vi "LDVLinearStage.vi"() -> ()   [LabVIEW 2016]
uses:
  <vilib>/Instr/_visa.llb/VISA Configure Serial Port (Instr).vi
panel:
  out "Response":string
  in  "Stop":bool
  in  "Starting Distance (mm)":dbl
  in  "Total Distance (mm)":dbl
  in  "Change in Distance (mm)":dbl
  in  "Wait Time (s)":u32
  in  "Send Commands":bool
  in  "Extra Commands":string
  # "Relevant SCL Commands\n\nAC - Acceleration\nFL - Feed to Length\nFP - Feed to Position\nID - Immediate Distance\nIP - Immediate Position\nJS - Jog Speed\nSJ - Stop Jogging\nSK - Stop and Kill Buffer\nSP - Set Position\n  (SP0; set current motor             position at absolute zero)\nVE - Velocity"
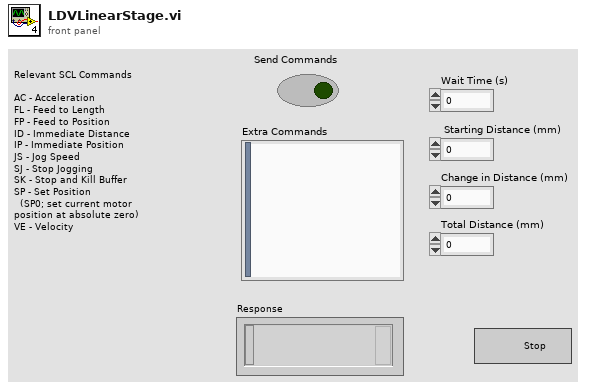
[diagram p1: front panel]
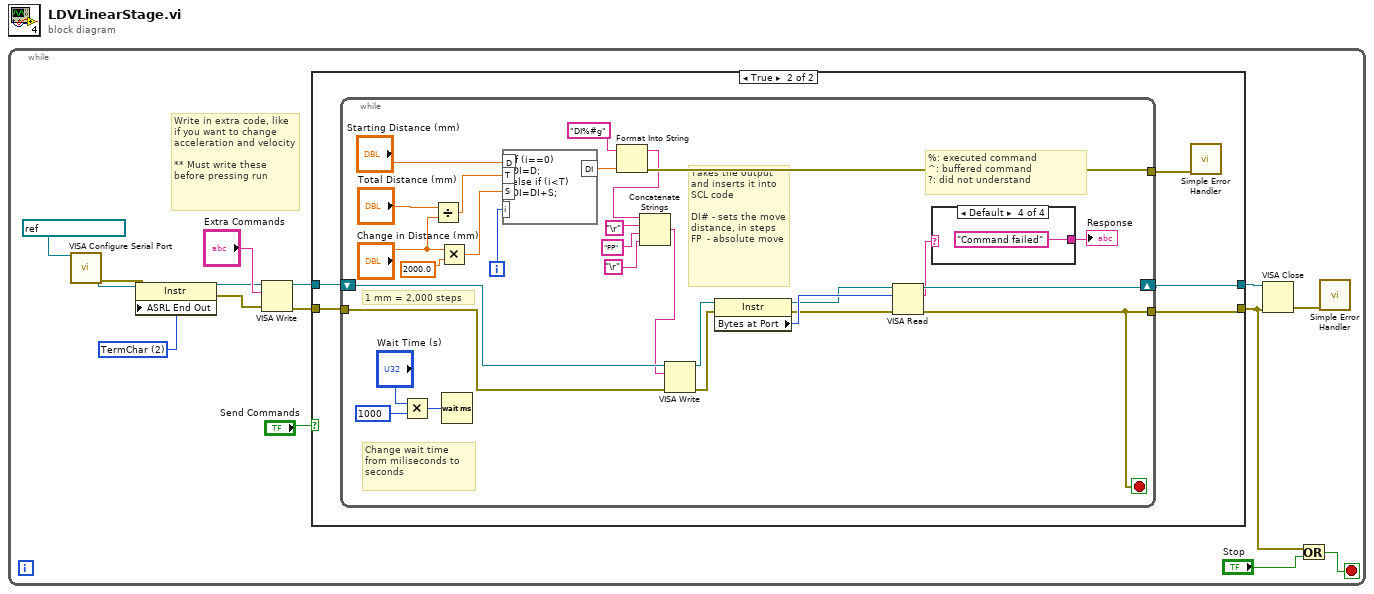
[diagram p0: block diagram]
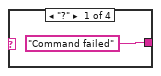
[diagram p3: hidden frame]
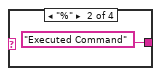
[diagram p4: hidden frame]
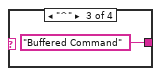
[diagram p5: hidden frame]
diagram:
  n1 = while {
    stop <- w1 stop-if-true
    w12 = u16 2 items=["None", "Last Bit", "TermChar", "Break"] ("Serial Settings:End Mode for Writes")
    # "Write in extra code, like if you want to change acceleration and velocity\n\n** Must write these before pressing run"
    n2 = call-poly "VISA Configure Serial Port"("VISA resource name"=refnum<visa-resource-name> "ASRL1::INSTR") -> ("VISA resource name out"=w14:refnum<visa-resource-name>, "error out"=w13:errorcluster)  [unwired: 13 in]
    n3 = property class="Instr"(reference=w14, error in=w13, "ASRL End Out"=w12) -> (reference out=w8:refnum<visa-resource-name>, error out=w7:errorcluster)
    n4 = VISA Write(VISA resource name=w8, write buffer="Extra Commands", error in (no error)=w7) -> (VISA resource name out=w5:refnum<visa-resource-name>, error out=w6:errorcluster)  [unwired: 1 out]
    n5 = case shown="True" "Send Commands" {
      tunnel: [w17 w18] -> w3
      tunnel: [w16 w22] -> w10
      tunnel: w6 -> [w17 w21]
      tunnel: w5 -> [w16 w20]
      frame False {
      }
      frame True {
        n6 = while {
          shift-right: [w28] -> w22
          shift-left: w20 -> [w49]
          tunnel: w21 -> [w51]
          tunnel: [w39] -> w19
          tunnel: [w23] -> w18
          i -> [w48]
          stop <- w23 stop-if-true
          # "%: executed command\n^: buffered command\n?: did not understand"
          # "Takes the output and inserts it into SCL code\n\nDI# - sets the move distance, in steps\nFP  - absolute move"
          # "Change wait time from miliseconds to seconds"
          # "1 mm = 2,000 steps"
          n7 = Multiply(x="Wait Time (s)", y=u32 1000) -> (x*y=w24:u32)
          n8 = Divide(x="Total Distance (mm)", y="Change in Distance (mm)") -> (x/y=w44:dbl)
          n9 = Multiply(x="Change in Distance (mm)", y=2000.0) -> (x*y=w45:dbl)
          n10 = Wait (ms)(milliseconds to wait=w24) -> ()  [unwired: 1 out]
          n11 = formula code="if (i==0)\nDI=D;\nelse if (i<T)\nDI=DI+S;"("D"="Starting Distance (mm)", "T"=w44, "S"=w45, "i"=w48) -> ("DI"=w42:dbl)
          n12 = Format Into String(format string="DI%#g", w42) -> (resulting string=w38:string, error out=w39:errorcluster)  [unwired: 2 in]
          n13 = Concatenate Strings(w38, "\r", "FP" ("string"), "\r") -> (w34:string)
          n14 = VISA Write(VISA resource name=w49, write buffer=w34, error in (no error)=w51) -> (VISA resource name out=w50:refnum<visa-resource-name>, error out=w40:errorcluster)  [unwired: 1 out]
          n15 = property class="Instr"(reference=w50, error in=w40) -> (reference out=w29:refnum<visa-resource-name>, error out=w30:errorcluster, "Bytes at Port"=w31:u32)
          n16 = VISA Read(VISA resource name=w29, byte count=w31, error in (no error)=w30) -> (VISA resource name out=w28:refnum<visa-resource-name>, read buffer=w27:string, error out=w23:errorcluster)  [unwired: 1 out]
          n17 = case shown="Default" w27 {
            tunnel: ["Command failed" "Executed Command" "Buffered Command" "Command failed"] -> w32
            frame "?" {
            }
            frame "%" {
            }
            frame "^" {
            }
            frame Default {
            }
          }
          "Response" <- w32
        }
        n18 = call <vilib>:"Simple Error Handler.vi"("error in (no error)"=w19) -> ()  [unwired: 1 in, 8 out]
      }
    }
    n19 = VISA Close(VISA resource name=w10, error in (no error)=w3) -> (error out=w11:errorcluster)
    n20 = Or(x=w3, y="Stop") -> (x .or. y?=w1:bool)
    n21 = call <vilib>:"Simple Error Handler.vi"("error in (no error)"=w11) -> ()  [unwired: 1 in, 8 out]
  }
